vi "niRFSTS SG Trim Invalid Characters.vi"(8 "error in (no error)":errorcluster, 11 "Waveform Name In":string="test") -> (0 "error out":errorcluster, 3 "Waveform Name Out":string="test")   [LabVIEW 2014]
doc: "Trim invalid characters from waveform name."
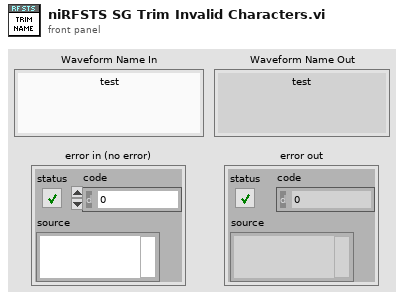
[diagram p1: front panel]
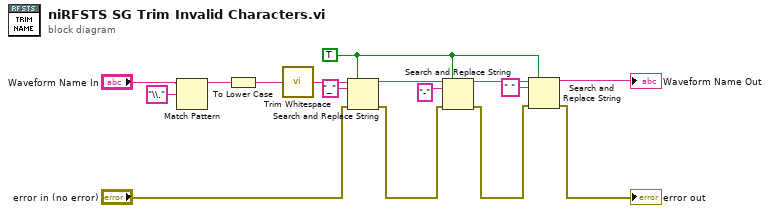
[diagram p0: block diagram]
diagram:
  w6 = TRUE ("replace all? (F)")
  n1 = Match Pattern(string="Waveform Name In", regular expression="\\.") -> (before substring=w2:string)  [unwired: 1 in, 3 out]
  n2 = To Lower Case(string=w2) -> (all lower case string=w1:string)
  n3 = call <vilib>:"Trim Whitespace.vi"("string"=w1) -> ("trimmed string"=w16:string)  [unwired: 1 in]
  n4 = Search and Replace String(replace all?=w6, input string=w16, search string="_", error in="error in (no error)") -> (result string=w13:string, error out=w9:errorcluster)  [unwired: 4 in, 2 out]
  n5 = Search and Replace String(replace all?=w6, input string=w13, search string="-", error in=w9) -> (result string=w11:string, error out=w8:errorcluster)  [unwired: 4 in, 2 out]
  n6 = Search and Replace String(replace all?=w6, input string=w11, search string=" ", error in=w8) -> (result string=→"Waveform Name Out":string, error out=→"error out":errorcluster)  [unwired: 4 in, 2 out]
